vi "Test 6.vi"   [LabVIEW 2021, in "Memory Map.lvclass"]
uses:
  Memory Map.lvclass
  Active Device.ctl
  <vilib>/addons/_JKI Toolkits/Caraya/classes/Assert/Assert Equal Value_Variant.vi
  <vilib>/addons/_JKI Toolkits/Caraya/classes/Test/Test.lvclass
  <vilib>/addons/_JKI Toolkits/Caraya/classes/Assert/Assert.lvclass
types:
  T1 = typedef "Memory Map.lvclass/Active Device.ctl" = enum16{"Error", "None", "RAM", "EEPROM", "VIA"}
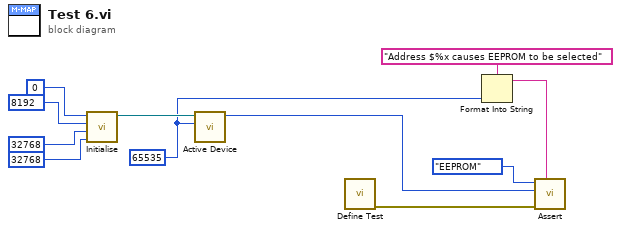
[diagram p0: block diagram]
diagram:
  w3 = u16 65535 ("RAM Base Address")
  n1 = call "Initialise.vi"("EEPROM Size"=u16 32768 ("RAM Base Address"), "EEPROM Base Address"=u16 32768 ("RAM Base Address"), "RAM Size"=u16 8192 ("RAM Base Address"), "RAM Base Address"=u16 0) -> ("Memory Map out"=w7:refnum<class "Memory Map.lvclass">)  [unwired: 7 in]
  n2 = call "Active Device.vi"("Address"=w3, "Memory Map in"=w7) -> ("Active Device"=w1:T1)  [unwired: 8 in, 1 out]
  n3 = call <vilib>:"Define Test.vi"() -> ("error out"=w6:errorcluster)  [unwired: 11 in]
  n4 = Format Into String(format string="Address $%x causes EEPROM to be selected" ("Label"), w3) -> (resulting string=w4:string)  [unwired: 2 in, 1 out]
  n5 = call-poly <vilib>:"Assert.vi"("Label"=w4, "error in (no error)"=w6, "Y"=w1, "X"=Active_Device."EEPROM" ("Active Device")) -> ()  [unwired: 7 in, 1 out]
